vi "SECoP_dataToJSON.vi"(8 "error in (no error)":errorcluster, 10 "SECoP_dataPtr":T1 {"ptr64" format="%.0x"; "ptr32" format="%.0x"}, 11 "DLL path (in)":T2) -> (0 "error out":errorcluster, 2 "JSONBuffer":string, 3 "DLL path (out)":T2)   [LabVIEW 2023, in "SECoP.lvlib"]
doc: "Call <b>\"SECoP_dataToJSON.vi\"</b> \n\n\nto create a SECoP command inside the last created SECoP module.\n\n<b>DLL path</b> input and output of cluster from \"SECoP-Initialize.vi\"\n<b>command name</b> name of command\n<b>datainfo</b> data info (data type of command, see SECoP specification)\n<b>description</b> human readable description of this command"
uses:
  SECoP.lvlib
  SECoP-libraries.ctl
  SECoP-data.ctl
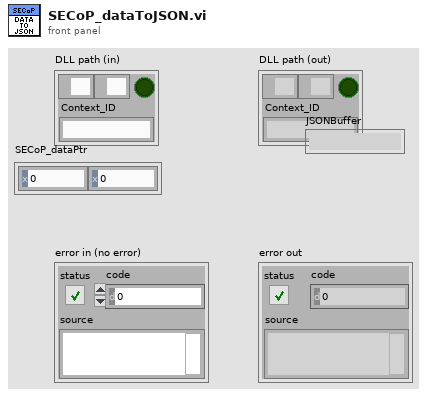
[diagram p1: front panel]
types:
  T1 = typedef "SECoP.lvlib/SECoP-data.ctl" = cluster{"ptr32":u32, "ptr64":u64}
  T2 = typedef "SECoP.lvlib/SECoP-libraries.ctl" = cluster{"serverDLL":path, "variantDLL":path, "cleanup_mode":bool, "Context_ID":string}
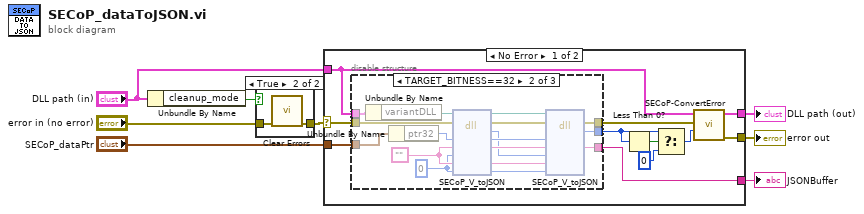
[diagram p0: block diagram]
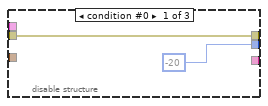
[diagram p3: hidden frame]
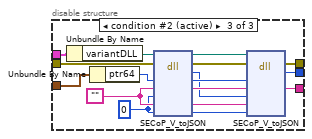
[diagram p4: hidden frame]
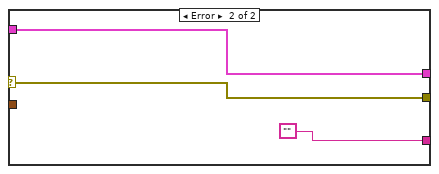
[diagram p5: hidden frame]
diagram:
  n1 = Unbundle By Name("DLL path (in)") -> ("cleanup_mode"=w5:bool)
  n2 = case shown="True" w5 {
    tunnel: "error in (no error)" -> [w9 w11]
    tunnel: [w9 w10] -> w3
    frame False {
    }
    frame True {
      n3 = call <vilib>:"Clear Errors.vi"("error in (no error)"=w11) -> ("error out"=w10:errorcluster)  [unwired: 5 in, 1 out]
    }
  }
  n4 = case shown="No Error" w3 {
    selector: w3 -> [w20 w60]
    tunnel: "DLL path (in)" -> [w12 w61]
    tunnel: [w21 w61] -> w7
    tunnel: [w22 w60] -> w6
    tunnel: [w14 ""] -> w2
    tunnel: "SECoP_dataPtr" -> [w13 _]
    frame No Error {
      n5 = disable-structure shown="TARGET_BITNESS==32" {
        disable-tunnel: w20 -> [w24 w40 w57]
        disable-tunnel: w12 -> [_ w39 w56]
        disable-tunnel: [w24 w25 w44] -> w19
        disable-tunnel: [-20 w26 w43] -> w17
        disable-tunnel: [_ w27 w42] -> w14
        disable-tunnel: w13 -> [_ w38 w55]
        frame condition #0 {
        }
        frame condition #1 {
          w41 = ""
          w35 = 0 ("BufferSize")
          n6 = Unbundle By Name(w39) -> ("variantDLL"=w36:path)
          n7 = Unbundle By Name(w38) -> ("ptr32"=w37:u32)
          n8 = dll-call lib="Z:/Praktische_Aufgaben/SECoP-LabVIEW2015/32bit/SECoP32.dll" fn="SECoP_V_toJSON"(path in=w36, error in=w40, "data"=w37, "JSONBuffer"=w41, "BufferSize"=w35, "PartBuffer"=w41, "PartBufferSize"=w35) -> (path out=w34:path, error out=w33:errorcluster, "return type"=w30:i32, "data"=w32:u32, "JSONBuffer"=w31:string, "PartBuffer"=w29:string, "PartBufferSize"=w28:i32)  [unwired: 2 in]
          n9 = dll-call lib="Z:/Praktische_Aufgaben/SECoP-LabVIEW2015/32bit/SECoP32.dll" fn="SECoP_V_toJSON"(path in=w34, error in=w33, "data"=w32, "JSONBuffer"=w31, "BufferSize"=w30, "PartBuffer"=w29, "PartBufferSize"=w28) -> (error out=w25:errorcluster, "return type"=w26:i32, "JSONBuffer"=w27:string)  [unwired: 5 in, 1 out]
        }
        frame condition #2 (active) {
          w58 = ""
          w52 = 0 ("BufferSize")
          n10 = Unbundle By Name(w56) -> ("variantDLL"=w53:path)
          n11 = Unbundle By Name(w55) -> ("ptr64"=w54:u64)
          n12 = dll-call lib="Z:/Praktische_Aufgaben/SECoP-LabVIEW2015/32bit/SECoP32.dll" fn="SECoP_V_toJSON"(path in=w53, error in=w57, "data"=w54, "JSONBuffer"=w58, "BufferSize"=w52, "PartBuffer"=w58, "PartBufferSize"=w52) -> (path out=w51:path, error out=w50:errorcluster, "return type"=w47:i32, "data"=w49:u64, "JSONBuffer"=w48:string, "PartBuffer"=w46:string, "PartBufferSize"=w45:i32)  [unwired: 2 in]
          n13 = dll-call lib="Z:/Praktische_Aufgaben/SECoP-LabVIEW2015/32bit/SECoP32.dll" fn="SECoP_V_toJSON"(path in=w51, error in=w50, "data"=w49, "JSONBuffer"=w48, "BufferSize"=w47, "PartBuffer"=w46, "PartBufferSize"=w45) -> (error out=w44:errorcluster, "return type"=w43:i32, "JSONBuffer"=w42:string)  [unwired: 5 in, 1 out]
        }
      }
      n14 = Less Than 0?(x=w17) -> (x < 0?=w18:bool)
      n15 = Select(t=w17, s=w18, f=0) -> (s? t:f=w16:i32)
      n16 = call "SECoP-ConvertError.vi"("return code"=w16, "error in (no error)"=w19, "DLL path (in)"=w12) -> ("error out"=w22:errorcluster, "DLL path (out)"=w21:T2)  [unwired: 7 in]
    }
    frame Error {
    }
  }
  "DLL path (out)" <- w7
  "error out" <- w6
  "JSONBuffer" <- w2
